vi "Insert Piece.vi"(8 "error in (no error)":errorcluster, 11 "Game Engine in":refnum<class "Game Engine.lvclass">) -> (0 "error out":errorcluster, 3 "Game Engine out":refnum<class "Game Engine.lvclass">)   [LabVIEW 2017, in "Game Engine.lvlib" / "Game Engine.lvclass"]
uses:
  Game Engine.lvclass
  Game Engine.lvclass/Game Engine.ctl
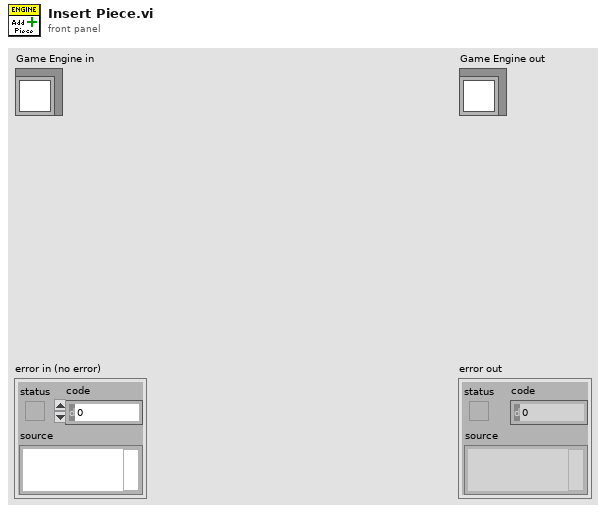
[diagram p1: front panel]
types:
  T1 = typedef "Game Engine.lvlib/Game Engine.lvclass/Piece.ctl" = u32[][]
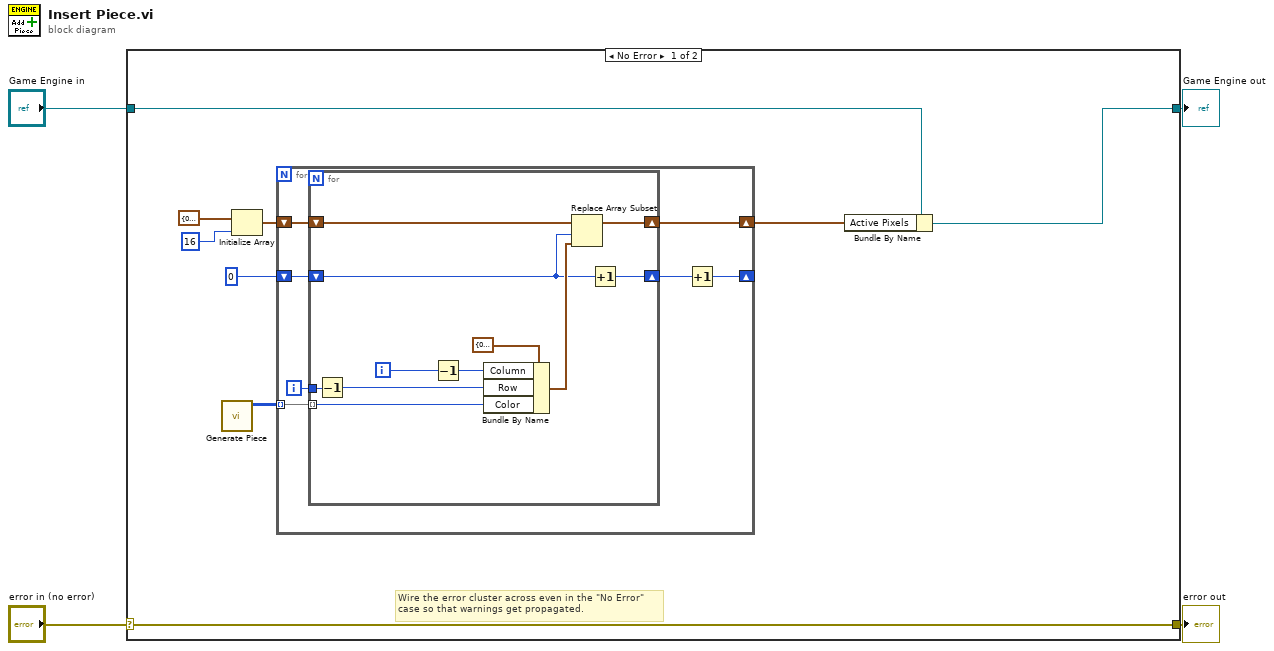
[diagram p0: block diagram]
diagram:
  n1 = case shown="No Error" "error in (no error)" {
    selector: "error in (no error)" -> [w13 w33]
    tunnel: [w13 w33] -> w3
    tunnel: [w6 w32] -> w1
    tunnel: "Game Engine in" -> [w7 w32]
    frame No Error {
      # "Wire the error cluster across even in the \"No Error\"\ncase so that warnings get propagated."
      n2 = call "Generate Piece.vi"() -> ("Piece"=w12:T1)  [unwired: 11 in]
      n3 = Initialize Array(cluster{"Column":u8, "Row":u8, "Color":u32} {"Column"=0, "Row"=0, "Color"=0} ("Active Piece Pixels"), 16 ("dimension size")) -> (w9:cluster{"Column":u8, "Row":u8, "Color":u32}[])
      n4 = for {
        tunnel: w12 -> [w18] mode=indexing
        shift-right: [w17] -> w8
        shift-left: w9 -> [w20]
        shift-right: [w14] -> _
        shift-left: 0 -> [w16]
        i -> [w19]
        n5 = for {
          shift-right: [w23] -> w17
          shift-left: w20 -> [w30]
          tunnel: w19 -> [w31]
          tunnel: w18 -> [w25] mode=indexing
          shift-right: [w21] -> w15
          shift-left: w16 -> [w22]
          i -> [w28]
          n6 = Decrement(x=w31) -> (x-1=w27:i32)
          n7 = Decrement(x=w28) -> (x-1=w26:i32)
          n8 = Bundle By Name(cluster=cluster{"Column":u8, "Row":u8, "Color":u32} {"Column"=0, "Row"=0, "Color"=0} ("Active Piece Pixels"), "Column"=w26, "Row"=w27, "Color"=w25) -> (w24:cluster{"Column":u8, "Row":u8, "Color":u32})
          n9 = Replace Array Subset(array=w30, new element=w24, index=w22) -> (w23:cluster{"Column":u8, "Row":u8, "Color":u32}[])
          n10 = Increment(x=w22) -> (x+1=w21:i32)
        }
        n11 = Increment(x=w15) -> (x+1=w14:i32)
      }
      n12 = Bundle By Name(cluster=w7, "Active Pixels"=w8) -> (w6:refnum<class "Game Engine.lvclass">)
    }
    frame Error {
    }
  }
  "error out" <- w3
  "Game Engine out" <- w1
